vi "Init FPGA Wave Generator.vi"(8 "error in":errorcluster, 10 "FPGA VI Reference In":refnum<k20>, 11 "Wave path":path) -> (3 "Done":bool=TRUE)   [LabVIEW 2014]
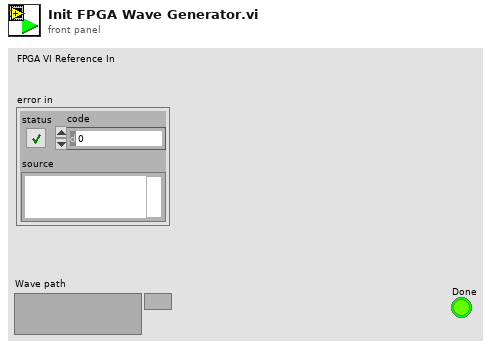
[diagram p1: front panel]
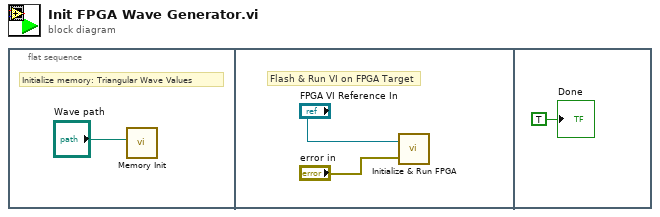
[diagram p0: block diagram]
diagram:
  n1 = flat-sequence {
    frame #0 {
      # "Initialize memory: Triangular Wave Values"
      n2 = call "Memory Init.vi"("Wave path"="Wave path") -> ()  [unwired: 9 in]
    }
    frame #1 {
      # "Flash & Run VI on FPGA Target"
      n3 = call "Initialize & Run FPGA.vi"("error in"="error in", "FPGA VI Reference In"="FPGA VI Reference In") -> ()  [unwired: 2 out]
    }
    frame #2 {
      "Done" <- TRUE
    }
  }
